vi "Get Module ID.vi"(8 "error in (no error)":errorcluster, 11 "GenNet Protocol in":refnum<class "GenNet Protocol.lvclass">) -> (0 "error out":errorcluster, 2 "Module ID":i32=-1, 3 "GenNet Protocol out":refnum<class "GenNet Protocol.lvclass">)   [LabVIEW 2020, in "hse-gennet.lvlib" / "GenNet Protocol.lvclass"]
doc: "____\nHAMPEL SOFTWARE ENGINEERING v3.8.0 (2023-12-18 14:41)"
uses:
  GenNet Protocol.lvclass
  GenNet Protocol.lvclass/GenNet Protocol.ctl
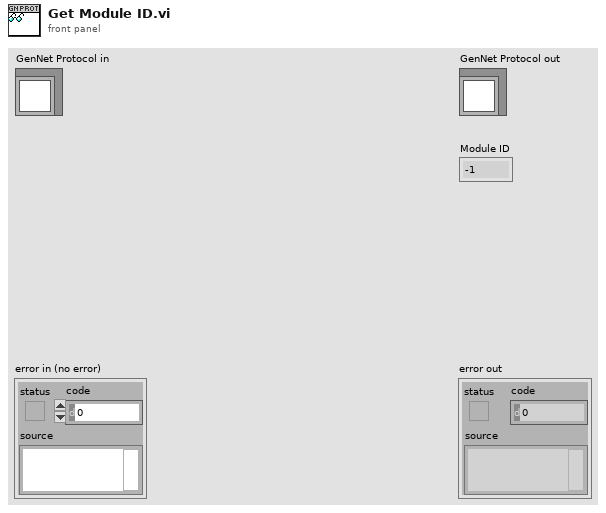
[diagram p1: front panel]
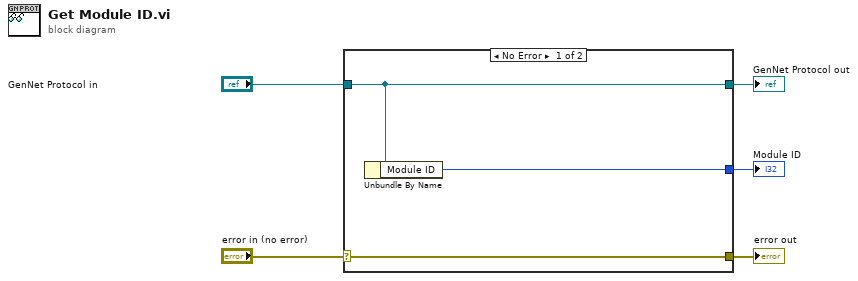
[diagram p0: block diagram]
diagram:
  n1 = case shown="No Error" "error in (no error)" {
    selector: "error in (no error)" -> [w8 w9]
    tunnel: [w8 w9] -> w4
    tunnel: [w7 w10] -> w2
    tunnel: "GenNet Protocol in" -> [w7 w10]
    tunnel: [w6 _] -> w1
    frame No Error {
      n2 = Unbundle By Name(w7) -> ("Module ID"=w6:i32)
    }
    frame Error {
    }
  }
  "error out" <- w4
  "GenNet Protocol out" <- w2
  "Module ID" <- w1
